vi "Jacobian Matrix 2 Diagonal.vi"(10 "Stiffness Jacobian In":T1=[[1000000.0, 0.0, 0.0, 0.0, 0.0, 0.0], [0.0, 1000000.0, 0.0, 0.0, 0.0, 0.0], [0.0, 0.0, 1000000.0, 0.0, 0.0, 0.0], [0.0, 0.0, 0.0, 1000000.0, 0.0, 0.0], [0.0, 0.0, 0.0, 0.0, 1000000.0, 0.0], [0.0, 0.0, 0.0, 0.0, 0.0, 1000000.0]]) -> (2 "Jacobian Diagonal Out":dbl[](array[numeric]))   [LabVIEW 2013]
uses:
  Stiffness Matrix.ctl
panel:
  # "dDx"
  # "dDy"
  # "dDz"
  # "dRx"
  # "dRy"
  # "dRz"
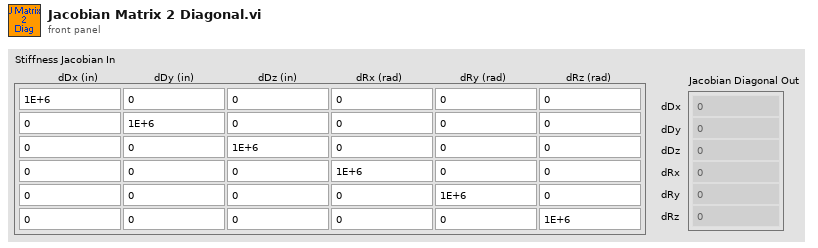
[diagram p1: front panel]
types:
  T1 = typedef "Stiffness Matrix.ctl" = dbl[][]
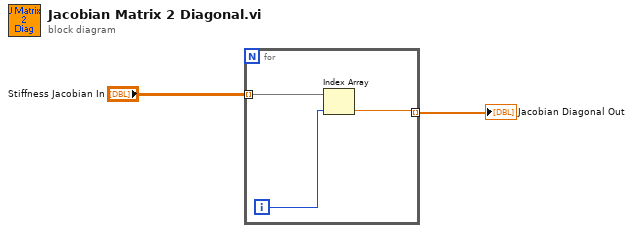
[diagram p0: block diagram]
diagram:
  n1 = for {
    tunnel: "Stiffness Jacobian In" -> [w5] mode=indexing
    tunnel: [w3] -> w1 mode=indexing
    i -> [w4]
    n2 = Index Array(array=w5, index=w4) -> (element=w3:dbl)
  }
  "Jacobian Diagonal Out" <- w1
